vi "Model Initial Values - Get Inport Channel Default.vi"(0 "error in":errorcluster, 3 "Item Ref in":T1 format="%.0x") -> (7 "error out":errorcluster, 9 "Default Value":dbl, 10 "Item Ref out":T1 format="%.0x")   [LabVIEW 2011, in "Model Initial Values Custom Device.lvlib"]
uses:
  Model Initial Values Custom Device.lvlib
  <vilib>/NI Veristand/Custom Device API/Custom Device Item Ref.ctl
  NationalInstruments.VeriStand.SystemStorage
  <vilib>/NI Veristand/Custom Device API/Custom Device API.lvlib
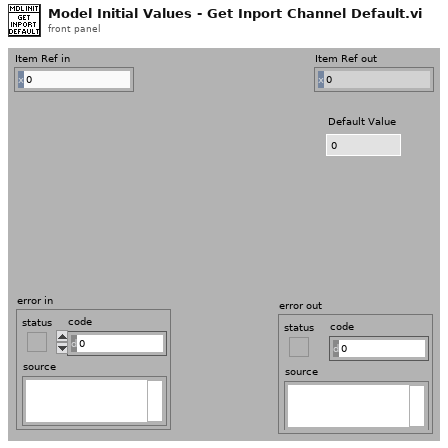
[diagram p1: front panel]
types:
  T1 = typedef "Custom Device API.lvlib/Custom Device Item Ref.ctl" = u64
  T2 = typedef "Custom Device API.lvlib/Custom Device Pointer.ctl" = refnum<k24>
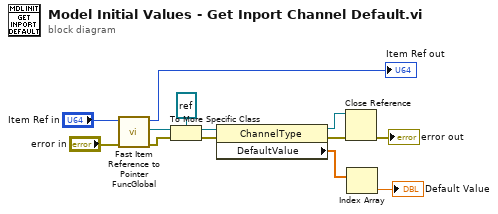
[diagram p0: block diagram]
diagram:
  n1 = call "Fast Item Reference to Pointer FuncGlobal.vi"("error in (no error)"="error in", "Item Ref in"="Item Ref in") -> ("error out"=w2:errorcluster, "Node Pointer"=w1:T2, "Item Ref out"=→"Item Ref out":T1)  [unwired: 6 in, 1 out]
  n2 = To More Specific Class(target class=refnum<k24> refnum ("BaseNodeType"), reference=w1, error in=w2) -> (specific class reference=w12:refnum<k24>, error out=w13:errorcluster)
  n3 = property class="ChannelType"(reference=w12, error in=w13) -> (reference out=w10:refnum<k24>, error out=w9:errorcluster, "DefaultValue"=w7:dbl[])
  n4 = Close Reference(reference=w10, error in (no error)=w9) -> (error out=→"error out":errorcluster)
  n5 = Index Array(array=w7) -> (element=→"Default Value":dbl)  [unwired: 1 in]
